vi "Peak.vi"(11 "POTTypedCircularBuffer in":refnum<class "ErrorLogBuffer.lvclass">) -> (2 "element":T1, 3 "POTTypedCircularBuffer out":refnum<class "ErrorLogBuffer.lvclass">)   [LabVIEW 2024, in "ErrorLogBuffer.lvclass"]
uses:
  ErrorLogBuffer.lvclass
  Type.ctl
  RQMHCore/ErrorReporting/Record/LogRecord.lvclass
  ErrorLogBuffer.lvclass/ErrorLogBuffer.ctl
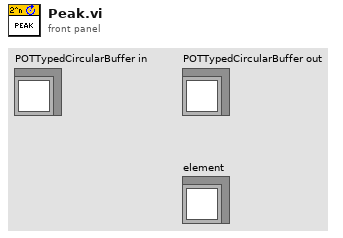
[diagram p1: front panel]
types:
  T1 = typedef "ErrorLogBuffer.lvclass/Type.ctl" = refnum<class "LogRecord.lvclass">
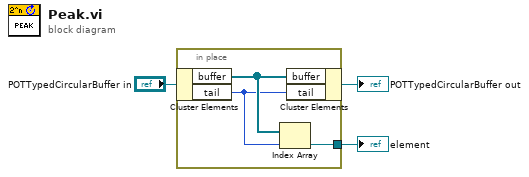
[diagram p0: block diagram]
diagram:
  n1 = in-place {
    in-place-border: [w5] -> w1
    n2 = in-place-cluster #1("POTTypedCircularBuffer in") -> ("buffer"=w6:T1[], "tail"=w4:i32)
    n3 = Index Array(array=w6, index=w4) -> (element=w5:T1)
    n4 = in-place-cluster #1("buffer"=w6, "tail"=w4) -> (→"POTTypedCircularBuffer out":refnum<class "ErrorLogBuffer.lvclass">)
  }
  "element" <- w1
